vi "ReadWait.vi"(8 "error in (no error)":errorcluster, 9 "Value":bool=TRUE, 10 "Read":i32, 11 "I-O in":refnum<class "I-O.lvclass">) -> (0 "error out":errorcluster, 3 "I-O out":refnum<class "I-O.lvclass">)   [LabVIEW 2016, in "I-O.lvclass"]
uses:
  I-O.lvclass
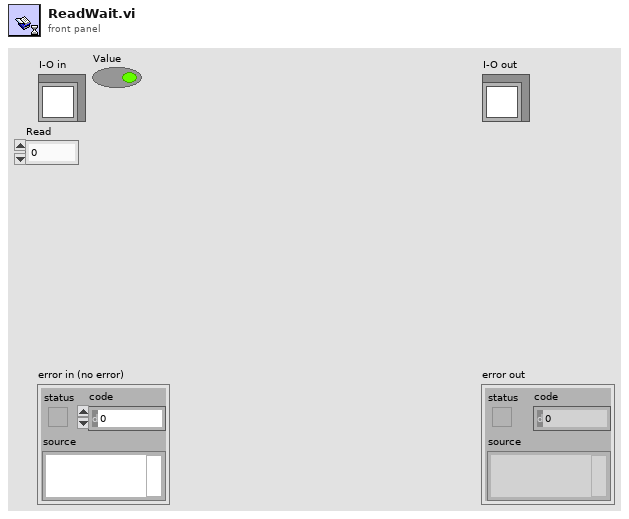
[diagram p1: front panel]
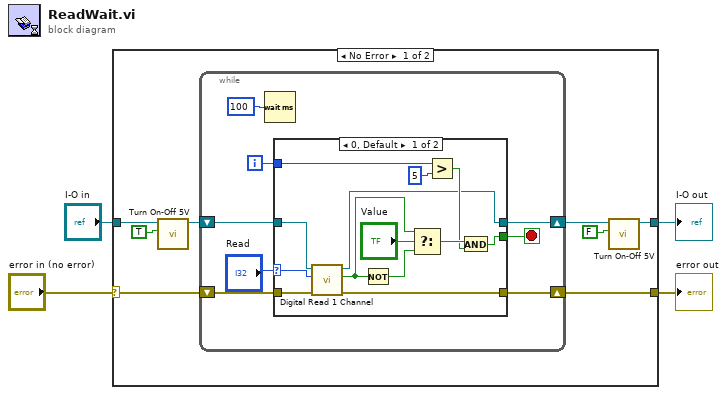
[diagram p0: block diagram]
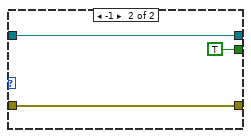
[diagram p2: hidden frame]
diagram:
  n1 = case shown="No Error" "error in (no error)" {
    selector: "error in (no error)" -> [w7 w38]
    tunnel: [w6 w38] -> w3
    tunnel: [w9 w37] -> w1
    tunnel: "I-O in" -> [w11 w37]
    frame No Error {
      n2 = call-dynamic "Turn On-Off 5V.vi"("Value"=TRUE, "I-O in"=w11) -> ("I-O out"=w8:refnum<class "I-O.lvclass">)  [unwired: 8 in, 1 out]
      n3 = while {
        shift-right: [w16] -> w5
        shift-left: w8 -> [w17]
        shift-right: [w14] -> w6
        shift-left: w7 -> [w15]
        i -> [w19]
        stop <- w18 stop-if-true
        n4 = Wait (ms)(milliseconds to wait=u32 100) -> ()  [unwired: 1 out]
        n5 = case shown="0, Default" "Read" {
          selector: "Read" -> [w22 _]
          tunnel: w19 -> [w32 _]
          tunnel: [w28 TRUE] -> w18
          tunnel: w17 -> [w27 w36]
          tunnel: [w25 w36] -> w16
          tunnel: w15 -> [w24 w34]
          tunnel: [w23 w34] -> w14
          frame 0, Default {
            n6 = call-dynamic "Digital Read 1 Channel.vi"("error in (no error)"=w24, "Read"=w22, "I-O in"=w27) -> ("error out"=w23:errorcluster, "Value"=w26:bool, "I-O out"=w25:refnum<class "I-O.lvclass">)  [unwired: 6 in]
            n7 = Not(x=w26) -> (.not. x?=w33:bool)
            n8 = Select(t=w26, s="Value", f=w33) -> (s? t:f=w30:bool)
            n9 = Greater?(x=w32, y=5) -> (0:w29:bool)
            n10 = And(x=w30, y=w29) -> (x .and. y?=w28:bool)
          }
          frame -1 {
          }
        }
      }
      n11 = call-dynamic "Turn On-Off 5V.vi"("Value"=FALSE, "I-O in"=w5) -> ("I-O out"=w9:refnum<class "I-O.lvclass">)  [unwired: 8 in, 1 out]
    }
    frame Error {
    }
  }
  "error out" <- w3
  "I-O out" <- w1
